vi "GetErrorStructureInnerWhitespace.vi"(8 "error in (no error)":errorcluster) -> (0 "error out":errorcluster, 3 "Case structure inner whitespace (px)":T1={"Left"=20, "Right"=20, "Top"=20, "Bottom"=40})   [LabVIEW 2017, in "ErrorStructureDrawer.lvlib"]
doc: "Gets the sizes of whitespacing to use between the inside of the case structure and its contents from the config FGV."
uses:
  ErrorStructureDrawer.lvlib
  Controls/CaseStructureInnerWhitespace.ctl
  Controls/GetSetCommand.ctl
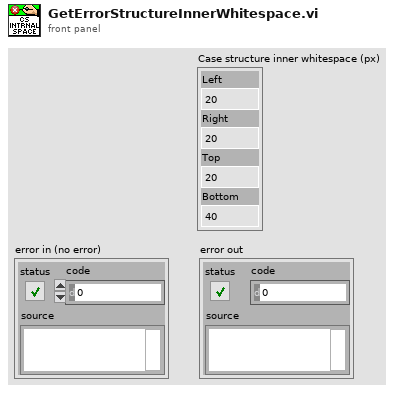
[diagram p1: front panel]
types:
  T1 = typedef "ErrorStructureDrawer.lvlib/CaseStructureInnerWhitespace.ctl" = cluster{"Left":u32, "Right":u32, "Top":u32, "Bottom":u32}
  T2 = typedef "ErrorStructureDrawer.lvlib/GetSetCommand.ctl" = enum16{"Get", "Set"}
  T3 = typedef "ErrorStructureDrawer.lvlib/ErrorStructureDrawerSettings.ctl" = cluster{"Error control config":T4, "BD alignment settings":T5, "Case structure outer whitespace (px)":T6, "Case structure inner whitespace (px)":T1, "Case structure constants":T7, "CS size if BD is empty":T8, "Control constants":T9}
  T4 = typedef "ErrorStructureDrawer.lvlib/ErrorControlConfig.ctl" = cluster{"Error control path":path, "Error indicator path":path, "Error control vertical spacing from existing FP items":i16, "Error-control to error-indicator horizontal spacing on FP":i16, "Error control vertical spacing from existing BD items":i32, "Error indicator vertical spacing from existing BD items":i32}
  T5 = typedef "ErrorStructureDrawer.lvlib/BD_AlignmentSettings.ctl" = cluster{"Controls":enum32{"Top Edges", "Vertical Centers", "Bottom Edges", "Left Edges", "Horizontal Centers", "Right Edges"}, "Indicators":enum32{"Top Edges", "Vertical Centers", "Bottom Edges", "Left Edges", "Horizontal Centers", "Right Edges"}}
  T6 = typedef "ErrorStructureDrawer.lvlib/CaseStructureOuterWhitespace.ctl" = cluster{"Control terminals right-side":i32, "Indicator terminals left-side":i32}
  T7 = typedef "ErrorStructureDrawer.lvlib/CaseStructureConstants.ctl" = cluster{"Border thickness":u32, "Case-menu height":u32, "Half height/width of a tunnel":i32}
  T8 = typedef "ErrorStructureDrawer.lvlib/CaseStructureSizeIfBD_Empty.ctl" = cluster{"Width (%)":dbl, "Height (%)":dbl}
  T9 = typedef "ErrorStructureDrawer.lvlib/ControlConstants.ctl" = cluster{"Half-height of terminal":i32}
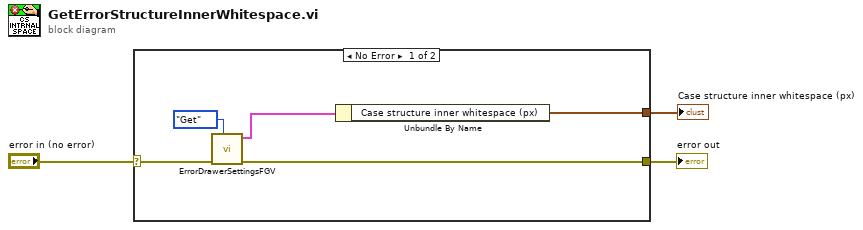
[diagram p0: block diagram]
diagram:
  n1 = case shown="No Error" "error in (no error)" {
    selector: "error in (no error)" -> [w5 w9]
    tunnel: [w8 w9] -> w3
    tunnel: [w4 _] -> w1
    frame No Error {
      n2 = call "ErrorDrawerSettingsFGV.vi"("Get or Set (Get)"=GetSetCommand."Get", "Error In"=w5) -> ("Error Out"=w8:errorcluster, "Error structure drawer settings"=w7:T3)  [unwired: 8 in]
      n3 = Unbundle By Name(w7) -> ("Case structure inner whitespace (px)"=w4:T1)
    }
    frame Error {
    }
  }
  "error out" <- w3
  "Case structure inner whitespace (px)" <- w1
